vi "Read IRs.vi"() -> (0 "Center":bool, 1 "Back":bool, 2 "Front":bool, 3 "Center raw":bool)   [LabVIEW 2013]
uses:
  Utilities/TimeManager.vi
  Common Code/Change Detect.vi
  Common Code/Change Detect Boolean.vi
  Robot Global Data.vi
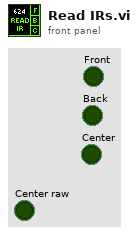
[diagram p1: front panel]
types:
  T1 = typedef "Dashboard UDP Packet.ctl" = cluster{"Camera":T2, "Gyro":T3, "Encoder":T5, "Auto Shift":T6, "Auton":T7, "Drive/Ramp X":dbl, "Drive/Ramp Y":dbl, "Drive/Battery Cutoff":dbl, "Pressure/Compressor Min Voltage":dbl, "Pressure/Compressor Delay":dbl, "Controller/Strafe Correction":bool, "Shooter":T8, "Rollers":T9, "Abort":bool, "Finish":bool}
  T2 = typedef "Camera Controls.ctl" = cluster{"Camera/View Angle X":dbl, "Camera/Goal Track Timeout":dbl, "Camera/View Angle Y":dbl, "Camera/Goal Exposure":dbl, "Camera/Vision Receive Timeout":dbl, "Camera/Offset 1":dbl, "Camera/Offset 2":dbl}
  T3 = typedef "Gyro Controls.ctl" = cluster{"Gyro/Angle Tolerance":dbl, "Gyro/Steer Closeness Threshold":dbl, "Steer PID":T4, "Steer Close PID":T4}
  T4 = typedef "PID Params.ctl" = cluster{"max":dbl, "min":dbl, "P":dbl, "I":dbl, "D":dbl}
  T5 = typedef "Encoder Controls.ctl" = cluster{"Encoders/Reset":bool, "Encoders/Omni Constant":dbl, "Encoders/Omni Tick Constant":dbl, "Encoders/Left Constant":dbl, "Encoders/Right Constant":dbl, "Encoders/Right Tick Constant":dbl}
  T6 = typedef "Auto Shift Controls.ctl" = cluster{"AutoShift/Upshift Throttle Accel":dbl, "AutoShift/Speed Threshold":dbl, "AutoShift/Upshift Throttle":dbl, "AutoShift/Upshift Accel":dbl, "AutoShift/Downshift Accel":dbl, "AutoShift/Downshift Throttle":dbl, "AutoShift/Delay":dbl, "AutoShift/Enabled":bool}
  T7 = typedef "Auton Controls.ctl" = cluster{"Auton/Left Shoot X-Coord":dbl, "Auton/Right Shoot X-Coord":dbl, "DistDrive/Distance Stop Threshold":dbl, "DistDrive/Max Stop Speed":dbl, "Auton/Back Piston Time":dbl, "Auton/Manual Hot":bool, "Auton/Manual Hot Right":bool, "Default X PID":T4, "Default Y PID":T4}
  T8 = typedef "Shooter Controls.ctl" = cluster{"Shooter/Reset Time":dbl, "Shooter/Release Delay":dbl, "Shooter/Pressure Steady Time":dbl, "Shooter/Misfire Delay":dbl, "Shooter/Ball Settle Time":dbl, "Shooter/Line IR Delay":dbl, "Pressure/Upper PSI Time":dbl, "Pressure/Lower PSI Time":dbl, "Shooter/Punch Delay":dbl, "Shooter/Target Pressure":dbl, "Pressure/Line B":dbl, "Pressure/Line M":dbl, "Pressure/Shooter M":dbl, "Pressure/Shooter B":dbl}
  T9 = typedef "Roller Controls.ctl" = cluster{"Roller/Load IRs Verify Time":dbl, "Roller/Center IR Latch Time":dbl, "Roller/Speed Front":dbl, "Roller/Speed Back":dbl, "Roller/Entry Timeout":dbl, "Roller/To Center Timeout":dbl, "Roller/Sustain Time":dbl, "Roller/Verify Center Time":dbl}
  T10 = typedef "WPI_DigitalInputDevRef.ctl" = cluster{"DevStatus":errorcluster, "DIO Channel":T11, "Digital Module":T12}
  T11 = typedef "FPGA_DIOChannel.ctl" = enum8{"DIO 1", "DIO 2", "DIO 3", "DIO 4", "DIO 5", "DIO 6", "DIO 7", "DIO 8", "DIO 9", "DIO 10", "DIO 11", "DIO 12", "DIO 13", "DIO 14", "Invalid"}
  T12 = typedef "FPGA_TypedefDigitalModule.ctl" = enum16{"Digital Module 1", "Digital Module 2"}
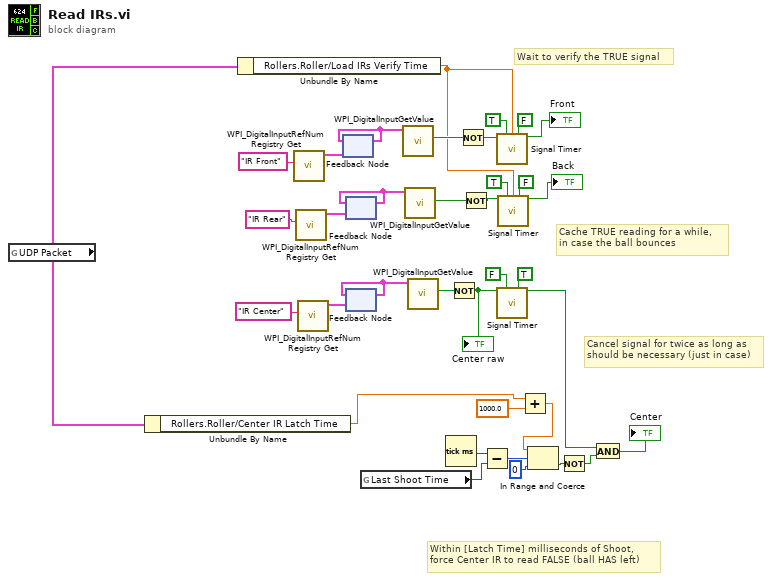
[diagram p0: block diagram]
diagram:
  # "Cancel signal for twice as long as\nshould be necessary (just in case)"
  # "Within [Latch Time] milliseconds of Shoot,\nforce Center IR to read FALSE (ball HAS left)"
  # "Wait to verify the TRUE signal"
  # "Cache TRUE reading for a while,\nin case the ball bounces"
  n1 = global read "Robot Global Data.vi" "UDP Packet"() -> (w2:T1)
  n2 = Unbundle By Name(w2) -> ("Rollers.Roller/Center IR Latch Time"=w1:dbl)
  n3 = Unbundle By Name(w2) -> ("Rollers.Roller/Load IRs Verify Time"=w3:dbl)
  n4 = call <vilib>:"WPI_DigitalInputRefNum Registry Get.vi"("refnum name"="IR Front") -> ("DigitalInputDevRef"=w34:T10)  [unwired: 9 in, 1 out]
  n5 = call <vilib>:"WPI_DigitalInputRefNum Registry Get.vi"("refnum name"="IR Rear") -> ("DigitalInputDevRef"=w32:T10)  [unwired: 9 in, 1 out]
  n6 = call <vilib>:"WPI_DigitalInputRefNum Registry Get.vi"("refnum name"="IR Center") -> ("DigitalInputDevRef"=w31:T10)  [unwired: 9 in, 1 out]
  n7 = feedback #1(w34) -> (w33:T10)
  n8 = feedback-in #1(w33) -> ()
  n9 = feedback #2(w32) -> (w29:T10)
  n10 = feedback-in #2(w29) -> ()
  n11 = feedback #3(w31) -> (w30:T10)
  n12 = feedback-in #3(w30) -> ()
  n13 = global read "Robot Global Data.vi" "Last Shoot Time"() -> (w16:u32)
  n14 = call <vilib>:"WPI_DigitalInputGetValue.vi"("DigitalInputDevRef"=w33) -> ("Value"=w27:bool)  [unwired: 8 in, 2 out]
  n15 = call <vilib>:"WPI_DigitalInputGetValue.vi"("DigitalInputDevRef"=w29) -> ("Value"=w26:bool)  [unwired: 8 in, 2 out]
  n16 = call <vilib>:"WPI_DigitalInputGetValue.vi"("DigitalInputDevRef"=w30) -> ("Value"=w28:bool)  [unwired: 8 in, 2 out]
  n17 = Tick Count (ms)() -> (millisecond timer value=w13:u32)
  n18 = Not(x=w28) -> (.not. x?=w25:bool)
  "Center raw" <- w25
  n19 = Not(x=w27) -> (.not. x?=w18:bool)
  n20 = Not(x=w26) -> (.not. x?=w17:bool)
  n21 = Subtract(x=w13, y=w16) -> (x-y=w15:u32)
  n22 = call "Signal Timer.vi"("Input"=w18, "Edge"=TRUE, "Interval"=w3, "Pull"=FALSE) -> ("Filtered Output"=→"Front":bool)  [unwired: 11 in]
  n23 = call "Signal Timer.vi"("Input"=w25, "Edge"=FALSE, "Pull"=TRUE) -> ("Filtered Output"=w10:bool)  [unwired: 12 in]
  n24 = call "Signal Timer.vi"("Input"=w17, "Edge"=TRUE, "Interval"=w3, "Pull"=FALSE) -> ("Filtered Output"=→"Back":bool)  [unwired: 11 in]
  n25 = Add(x=w1, y=1000.0) -> (x+y=w9:dbl)
  n26 = In Range and Coerce(upper limit=w9, x=w15, lower limit=u32 0) -> (In Range?=w12:bool)  [unwired: 1 out]
  n27 = Not(x=w12) -> (.not. x?=w11:bool)
  n28 = And(x=w10, y=w11) -> (x .and. y?=→"Center":bool)
